vi "Accurate Measure With Setting - 複製.vi"(0 "DMM ref in":refnum<visa-resource-name>, 1 "channel_count":i32=11, 2 "P_current_count":i32, 3 "N_current_count":i32, 5 "DMM error in":errorcluster, 7 "Accurate Measure Setting":T1, 9 "ESP32 ref in":refnum<visa-resource-name>, 11 "ESP32 error in":errorcluster, 12 "current_mode":u8[](array[numeric])=[0, 0, 0, 0, 0, 0, 0, 0, 0, 0, 0]) -> (4 "DMM ref out":refnum<visa-resource-name>, 6 "DMM error out":errorcluster, 8 "Accurate Data":dbl[](array[numeric]), 10 "ESP32 ref out":refnum<visa-resource-name>, 13 "time_out_count":i32, 14 "Standard Deviation of Data":dbl[](array[numeric]), 15 "ESP32 error out":errorcluster)   [LabVIEW 2023]
uses:
  <instrlib>/Agilent 3446X Series/Agilent 3446X Series.lvlib
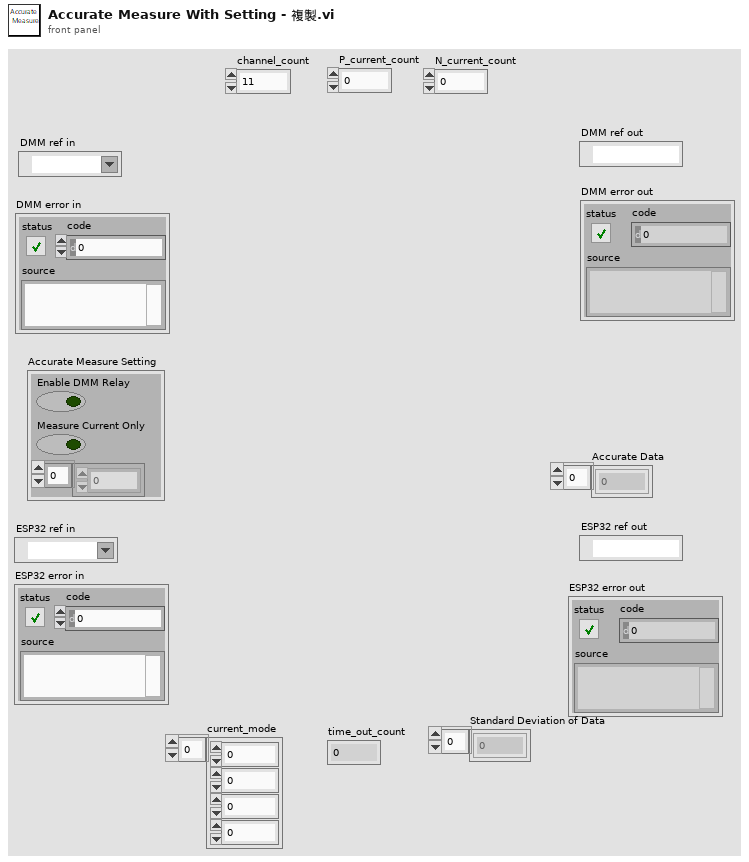
[diagram p1: front panel]
types:
  T1 = cluster{"Enable DMM Relay":bool, "Measure Current Only":bool, dbl[]}
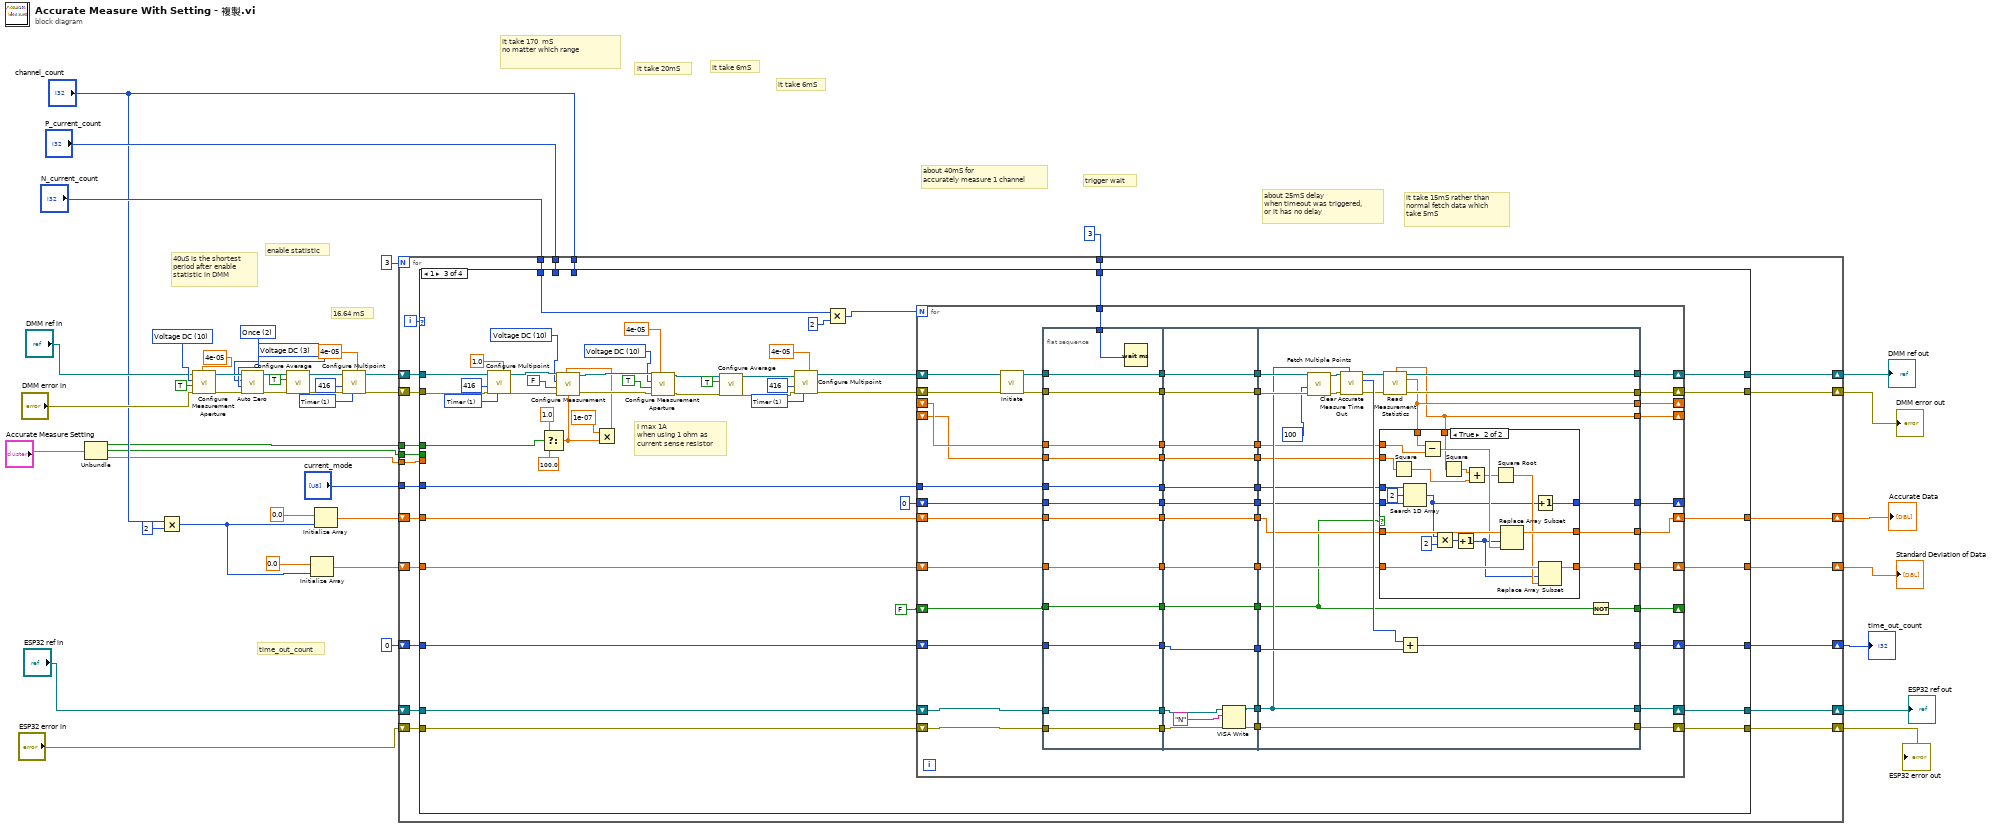
[diagram p0: block diagram]
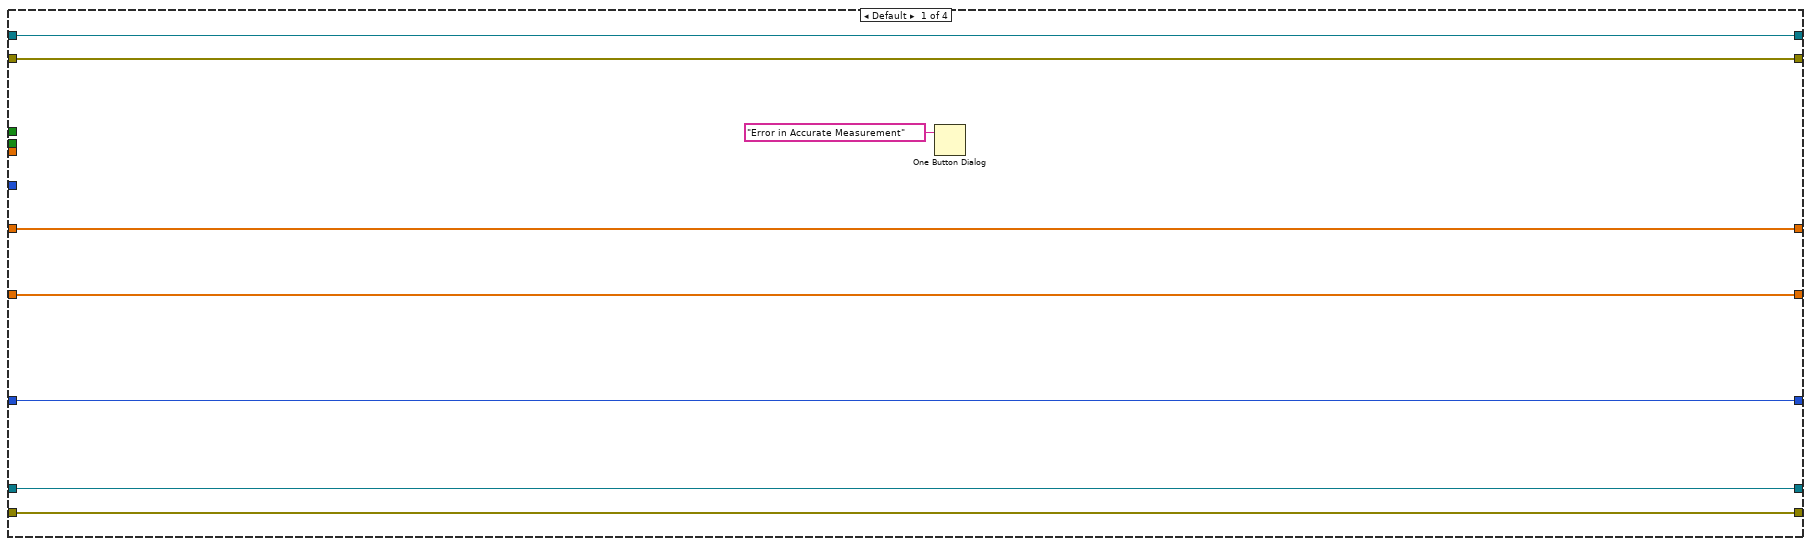
[diagram p2: hidden frame]
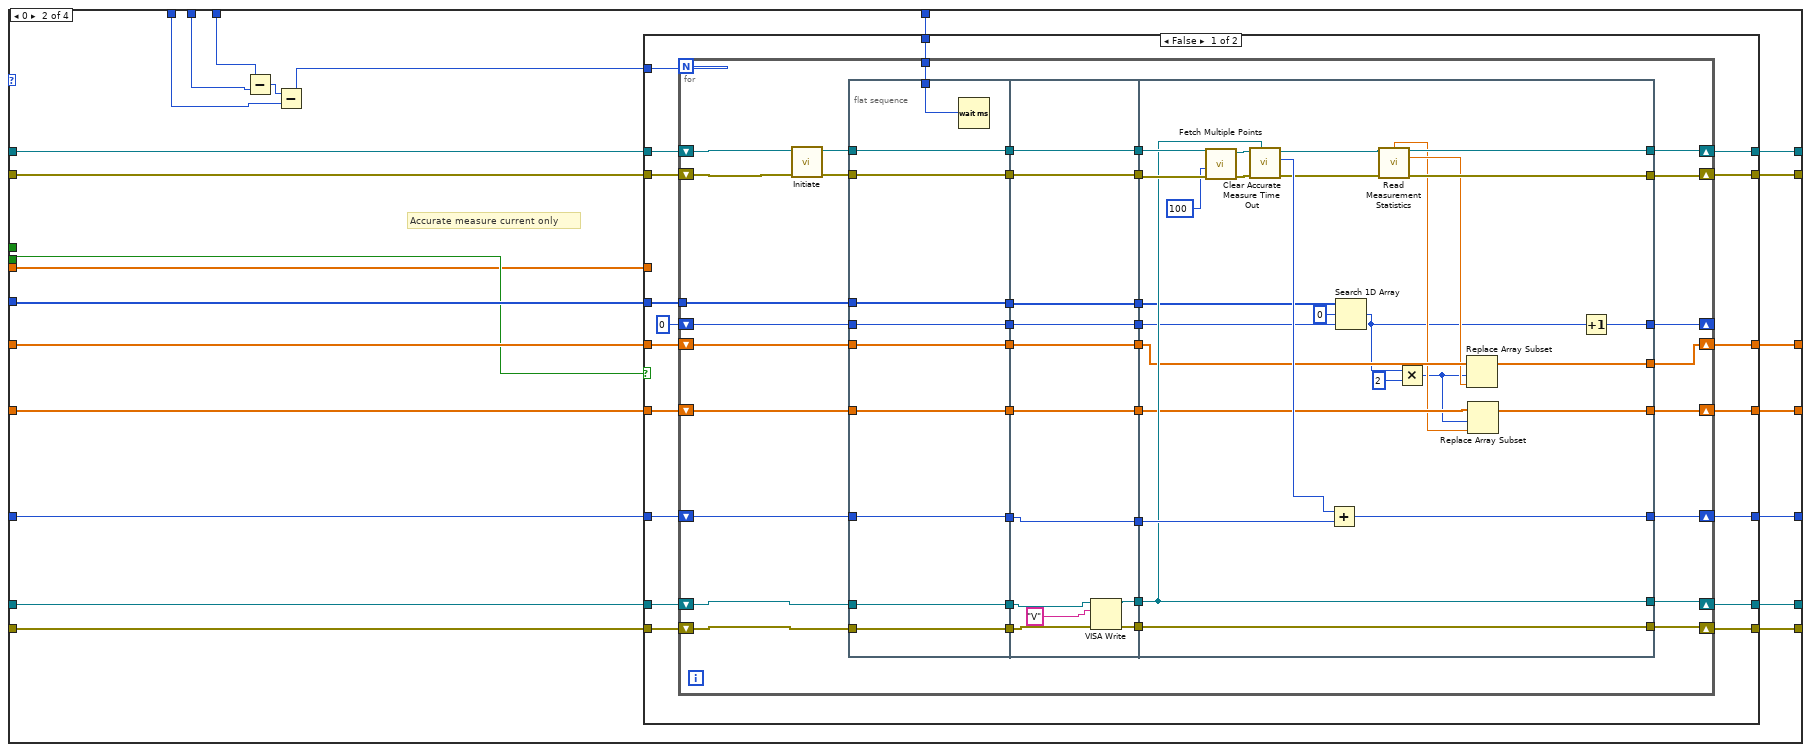
[diagram p3: hidden frame]
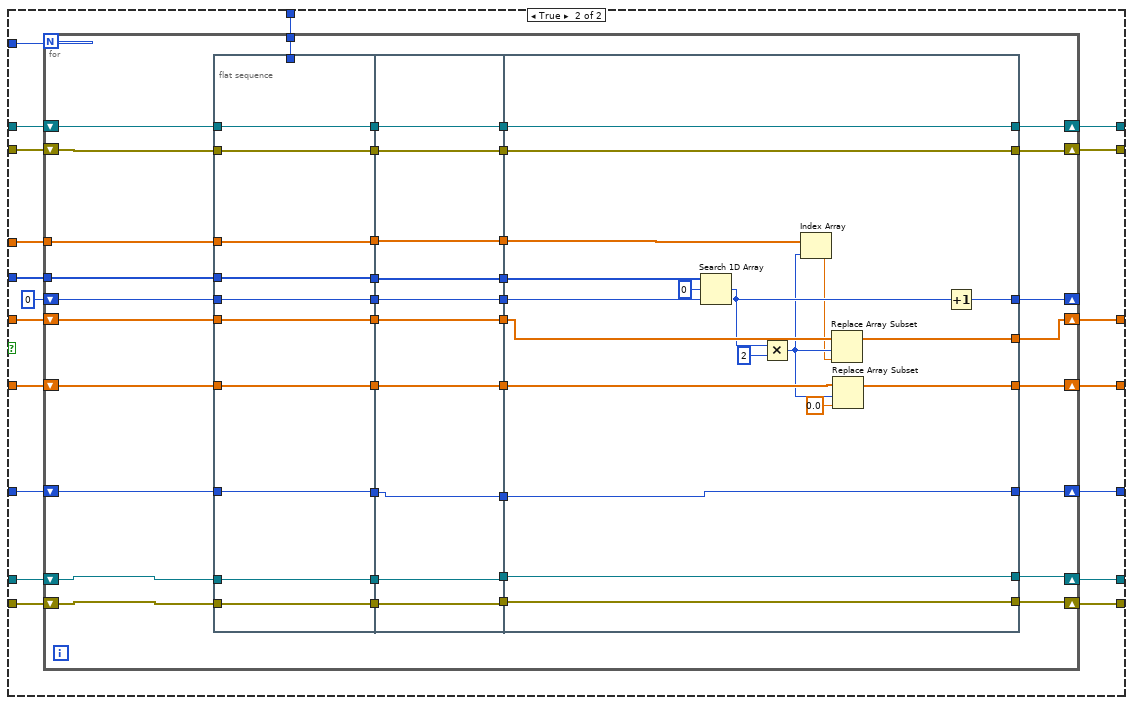
[diagram p4: hidden frame]
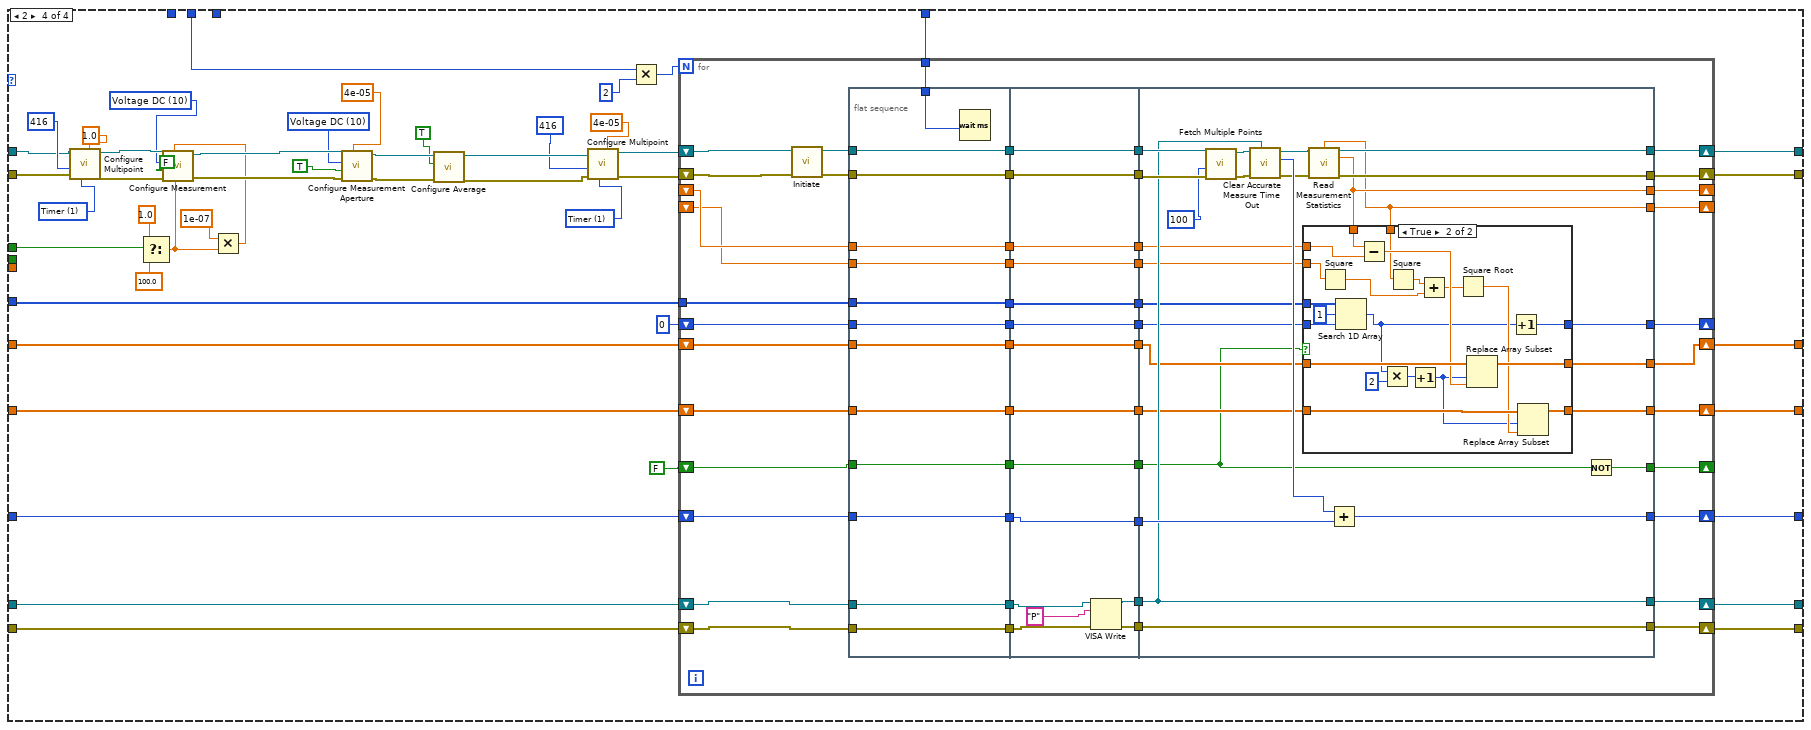
[diagram p6: hidden frame]
diagram:
  w32 = 1 items=["Immediate", "Timer"] ("Sample Source (0: Immediate)")
  w39 = 3 items=["Current DC", "Resistance", "Temperature", "Voltage DC"] ("Zero Type (0: Current DC)")
  w40 = 2 items=["Disable", "Enable", "Once"] ("Auto Zero (1: Enable)")
  w36 = 10 items=["Continuity", "Current AC", "Current DC", "Diode", "Frequency", "Resistance 4-wire", "Period", "Resistance 2-wire", "Temperature", "Voltage AC", "Voltage DC", "Voltage DC Ratio", "Capacitance"] ("Measurement Function (0: Continuity)")
  # "it take 6mS"
  # "it take 6mS"
  # "it take 20mS"
  # "it take 170  mS\nno matter which range"
  # "it take 15mS rather than\nnormal fetch data which \ntake 5mS"
  # "about 40mS for \naccurately measure 1 channel"
  # "about 25mS delay\nwhen timeout was triggered,\nor it has no delay"
  # "time_out_count"
  # "trigger wait"
  # "16.64 mS"
  # "enable statistic"
  # "40uS is the shortest\nperiod after enable \nstatistic in DMM"
  n1 = Unbundle("Accurate Measure Setting") -> ("Enable DMM Relay"=w4:bool, "Measure Current Only"=w2:bool, w1:dbl[])
  n2 = Multiply(x="channel_count", y=2) -> (x*y=w5:i32)
  n3 = call <instrlib>:"Configure Measurement Aperture.vi"("Aperture Time (0.1s)"=4e-05, "error in (no error)"="DMM error in", "Enable Aperture (F: Disable)"=TRUE, "Measurement Function (0: Continuity)"=w36, "VISA resource name"="DMM ref in") -> ("error out"=w43:errorcluster, "VISA resource name out"=w42:refnum<visa-resource-name>)  [unwired: 5 in]
  n4 = call <instrlib>:"Auto Zero.vi"("error in (no error)"=w43, "Auto Zero (1: Enable)"=w40, "Zero Type (0: Current DC)"=w39, "VISA resource name"=w42) -> ("error out"=w45:errorcluster, "VISA resource name out"=w44:refnum<visa-resource-name>)  [unwired: 6 in]
  n5 = call <instrlib>:"Configure Average.vi"("error in (no error)"=w45, "Enable Statistics (F: Disable)"=TRUE, "VISA resource name"=w44) -> ("error out"=w34:errorcluster, "VISA resource name out"=w35:refnum<visa-resource-name>)  [unwired: 7 in]
  n6 = Initialize Array(0.0 ("Arithmetic Mean"), w5) -> (w15:dbl[])
  n7 = Initialize Array(0.0 ("Arithmetic Mean"), w5) -> (w18:dbl[])
  n8 = call <instrlib>:"Configure Multipoint.vi"("Sample Interval (1 Second)"=4e-05, "Sample Source (0: Immediate)"=w32, "error in (no error)"=w34, "Sample Count (1)"=416, "VISA resource name"=w35) -> ("error out"=w29:errorcluster, "VISA resource name out"=w30:refnum<visa-resource-name>)  [unwired: 2 in, 3 out]
  n9 = for {
    N: 3 -> [_]
    shift-right: [w66] -> w11
    shift-left: "ESP32 ref in" -> [w68]
    shift-right: [w65] -> w10
    shift-left: "ESP32 error in" -> [w67]
    shift-right: [w62] -> w13
    shift-left: w30 -> [w64]
    shift-right: [w61] -> w12
    shift-left: w29 -> [w63]
    tunnel: "channel_count" -> [w60]
    tunnel: "P_current_count" -> [w59]
    tunnel: "N_current_count" -> [w58]
    tunnel: u32 3 ("milliseconds to wait") -> [w57]
    shift-right: [w56] -> w20
    shift-left: 0 -> [w55]
    shift-right: [w49] -> w9
    shift-left: w18 -> [w54]
    tunnel: "current_mode" -> [w53]
    shift-right: [w50] -> w8
    shift-left: w15 -> [w51]
    tunnel: w4 -> [w48]
    tunnel: w2 -> [w47]
    tunnel: w1 -> [w46]
    i -> [w52]
    n10 = case shown="1" w52 {
      tunnel: w68 -> [w74 w95 w350 w528]
      tunnel: w67 -> [w73 w94 w349 w527]
      tunnel: [w74 w91 w346 w524] -> w66
      tunnel: [w73 w90 w345 w523] -> w65
      tunnel: w64 -> [w76 w97 w314 w485]
      tunnel: w63 -> [w75 w96 w313 w484]
      tunnel: [w76 w93 w348 w526] -> w62
      tunnel: [w75 w92 w347 w525] -> w61
      tunnel: w60 -> [_ w89 _ _]
      tunnel: w59 -> [_ w88 _ w481]
      tunnel: w58 -> [_ w87 w309 _]
      tunnel: [w70 w85 w343 w521] -> w56
      tunnel: w57 -> [_ w86 w344 w522]
      tunnel: w55 -> [w70 w84 w342 w520]
      tunnel: w54 -> [w72 w82 w340 w518]
      tunnel: w53 -> [_ w83 w341 w519]
      tunnel: w51 -> [w71 w81 w338 w516]
      tunnel: [w71 w80 w337 w515] -> w50
      tunnel: [w72 w79 w336 w514] -> w49
      tunnel: w48 -> [_ _ w302 w486]
      tunnel: w47 -> [_ w78 _ _]
      tunnel: w46 -> [_ w77 _ _]
      frame Default {
        n11 = One Button Dialog(message="Error in Accurate Measurement") -> ()  [unwired: 1 in, 1 out]
      }
      frame 0 {
        # "Accurate measure current only"
        n12 = Subtract(x=w89, y=w88) -> (x-y=w99:i32)
        n13 = Subtract(x=w99, y=w87) -> (x-y=w98:i32)
        n14 = case shown="False" w78 {
          tunnel: w98 -> [w117 w223]
          tunnel: w97 -> [w116 w222]
          tunnel: w96 -> [w115 w221]
          tunnel: w95 -> [w114 w220]
          tunnel: w94 -> [w113 w219]
          tunnel: [w112 w218] -> w93
          tunnel: [w111 w217] -> w92
          tunnel: [w110 w216] -> w91
          tunnel: [w109 w215] -> w90
          tunnel: w86 -> [w108 w214]
          tunnel: [w107 w213] -> w85
          tunnel: w84 -> [w106 w212]
          tunnel: w83 -> [w105 w211]
          tunnel: w82 -> [w104 w210]
          tunnel: w81 -> [w102 w208]
          tunnel: [w101 w207] -> w80
          tunnel: [w100 w206] -> w79
          tunnel: w77 -> [_ w205]
          frame False {
            n15 = for {
              N: w117 -> [_]
              shift-right: [w151] -> w112
              shift-left: w116 -> [w155]
              shift-right: [w150] -> w111
              shift-left: w115 -> [w154]
              shift-right: [w149] -> w110
              shift-left: w114 -> [w153]
              shift-right: [w148] -> w109
              shift-left: w113 -> [w152]
              tunnel: w108 -> [w134]
              shift-right: [w133] -> w107
              shift-left: w106 -> [w147]
              tunnel: w105 -> [w131]
              shift-right: [w119] -> w100
              shift-left: w104 -> [w128]
              shift-right: [w123] -> _
              shift-left: 0 ("index of element") -> [w124]
              shift-right: [w118] -> w101
              shift-left: w102 -> [w121]
              n16 = call <instrlib>:"Initiate.vi"("error in (no error)"=w154, "VISA resource name"=w155) -> ("error out"=w135:errorcluster, "VISA resource name out"=w136:refnum<visa-resource-name>)  [unwired: 8 in]
              n17 = flat-sequence {
                tunnel: [w165] -> w146
                tunnel: w153 -> [w165]
                tunnel: [w164] -> w145
                tunnel: w152 -> [w164]
                tunnel: w136 -> [w163]
                tunnel: [w163] -> w144
                tunnel: [w162] -> w143
                tunnel: w135 -> [w162]
                tunnel: [w161] -> w142
                tunnel: w147 -> [w161]
                tunnel: w134 -> [w160]
                tunnel: [w159] -> w132
                tunnel: w131 -> [w159]
                tunnel: [w158] -> w129
                tunnel: w128 -> [w158]
                tunnel: w124 -> [w157]
                tunnel: [w157] -> w126
                tunnel: [w156] -> w122
                tunnel: w121 -> [w156]
                tunnel: w146 -> [w177]
                tunnel: w145 -> [w176]
                tunnel: w144 -> [w175]
                tunnel: [w175] -> w138
                tunnel: w143 -> [w174]
                tunnel: [w174] -> w139
                tunnel: [w173] -> w140
                tunnel: [w172] -> w141
                tunnel: w142 -> [w170]
                tunnel: [w170] -> w137
                tunnel: w132 -> [w169]
                tunnel: [w169] -> w130
                tunnel: w129 -> [w168]
                tunnel: [w168] -> w127
                tunnel: w126 -> [w167]
                tunnel: [w167] -> w125
                tunnel: w122 -> [w166]
                tunnel: [w166] -> w120
                tunnel: [w204] -> w148
                tunnel: [w192] -> w149
                tunnel: [w196] -> w150
                tunnel: [w197] -> w151
                tunnel: w141 -> [w204]
                tunnel: w140 -> [w192]
                tunnel: w139 -> [w203]
                tunnel: w138 -> [w202]
                tunnel: [w198] -> w133
                tunnel: w137 -> [w193]
                tunnel: w130 -> [w191]
                tunnel: w127 -> [w187]
                tunnel: w125 -> [w189]
                tunnel: [w188] -> w123
                tunnel: w120 -> [w185]
                tunnel: [w183] -> w119
                tunnel: [w182] -> w118
                frame #0 {
                  n18 = Wait (ms)(milliseconds to wait=w160) -> ()  [unwired: 1 out]
                }
                frame #1 {
                  n19 = VISA Write(VISA resource name=w177, write buffer="V" ("data in"), error in (no error)=w176) -> (VISA resource name out=w173:refnum<visa-resource-name>, error out=w172:errorcluster)  [unwired: 1 out]
                }
                frame #2 {
                  n20 = call <instrlib>:"Fetch Multiple Points.vi"("error in (no error)"=w203, "Timeout (10000 ms)"=100, "VISA resource name"=w202) -> ("error out"=w200:errorcluster, "VISA resource name out"=w201:refnum<visa-resource-name>)  [unwired: 1 in, 6 out]
                  n21 = call "Clear Accurate Measure Time Out.vi"("ESP32 ref"=w192, "error in (no error)"=w200, "DMM ref"=w201) -> ("error out"=w194:errorcluster, "Time out count"=w199:i32, "VISA Refnum out"=w195:refnum<visa-resource-name>)  [unwired: 5 in, 1 out]
                  n22 = Add(x=w199, y=w193) -> (x+y=w198:i32)
                  n23 = Search 1D Array(1D array=w191, element=u8 0, start index (0)=w189) -> (index of element=w180:i32)
                  n24 = call <instrlib>:"Read Measurement Statistics.vi"("VISA resource name"=w195, "error in (no error)"=w194) -> ("Standard Deviation"=w184:dbl, "VISA resource name out"=w197:refnum<visa-resource-name>, "Arithmetic Mean"=w186:dbl, "error out"=w196:errorcluster)  [unwired: 6 in, 4 out]
                  n25 = Multiply(x=w180, y=2) -> (x*y=w178:i32)
                  n26 = Replace Array Subset(array=w187, new element=w186, index=w178) -> (w183:dbl[])
                  n27 = Replace Array Subset(array=w185, new element=w184, index=w178) -> (w182:dbl[])
                  n28 = Increment(x=w180) -> (x+1=w188:i32)
                }
              }
            }
          }
          frame True {
            n29 = for {
              N: w223 -> [_]
              shift-right: [w232] -> w218
              shift-left: w222 -> [w234]
              shift-right: [w227] -> w217
              shift-left: w221 -> [w229]
              shift-right: [w260] -> w216
              shift-left: w220 -> [w262]
              shift-right: [w259] -> w215
              shift-left: w219 -> [w261]
              tunnel: w214 -> [w251]
              shift-right: [w250] -> w213
              shift-left: w212 -> [w258]
              tunnel: w211 -> [w248]
              shift-right: [w236] -> w206
              shift-left: w210 -> [w245]
              shift-right: [w240] -> _
              shift-left: 0 ("index of element") -> [w241]
              shift-right: [w235] -> w207
              shift-left: w208 -> [w238]
              tunnel: w205 -> [w224]
              n30 = flat-sequence {
                tunnel: [w272] -> w257
                tunnel: w262 -> [w272]
                tunnel: [w271] -> w256
                tunnel: w261 -> [w271]
                tunnel: [w270] -> w255
                tunnel: w258 -> [w270]
                tunnel: w251 -> [_]
                tunnel: [w269] -> w249
                tunnel: w248 -> [w269]
                tunnel: [w268] -> w246
                tunnel: w245 -> [w268]
                tunnel: w241 -> [w267]
                tunnel: [w267] -> w243
                tunnel: [w266] -> w239
                tunnel: w238 -> [w266]
                tunnel: w234 -> [w265]
                tunnel: [w265] -> w231
                tunnel: [w264] -> w230
                tunnel: w229 -> [w264]
                tunnel: [w263] -> w226
                tunnel: w224 -> [w263]
                tunnel: w257 -> [w275]
                tunnel: w256 -> [w274]
                tunnel: [w275] -> w253
                tunnel: [w274] -> w254
                tunnel: w255 -> [w282]
                tunnel: [w282] -> w252
                tunnel: w249 -> [w281]
                tunnel: [w281] -> w247
                tunnel: w246 -> [w280]
                tunnel: [w280] -> w244
                tunnel: w243 -> [w279]
                tunnel: [w279] -> w242
                tunnel: w239 -> [w278]
                tunnel: [w278] -> w237
                tunnel: [w277] -> w233
                tunnel: w231 -> [w277]
                tunnel: w230 -> [w276]
                tunnel: [w276] -> w228
                tunnel: w226 -> [w273]
                tunnel: [w273] -> w225
                tunnel: [w301] -> w259
                tunnel: [w300] -> w260
                tunnel: w254 -> [w301]
                tunnel: w253 -> [w300]
                tunnel: [w283] -> w250
                tunnel: w252 -> [w283]
                tunnel: w247 -> [w299]
                tunnel: w244 -> [w295]
                tunnel: w242 -> [w297]
                tunnel: [w296] -> w240
                tunnel: w237 -> [w294]
                tunnel: [w293] -> w236
                tunnel: [w292] -> w235
                tunnel: w233 -> [w289]
                tunnel: [w289] -> w232
                tunnel: [w288] -> w227
                tunnel: w228 -> [w288]
                tunnel: w225 -> [w286]
                frame #0 {
                }
                frame #1 {
                }
                frame #2 {
                  n31 = Search 1D Array(1D array=w299, element=u8 0, start index (0)=w297) -> (index of element=w291:i32)
                  n32 = Multiply(x=w291, y=2) -> (x*y=w285:i32)
                  n33 = Index Array(array=w286, index=w285) -> (element=w284:dbl)
                  n34 = Replace Array Subset(array=w295, new element=w284, index=w285) -> (w293:dbl[])
                  n35 = Replace Array Subset(array=w294, new element=0.0 ("new element/subarray"), index=w285) -> (w292:dbl[])
                  n36 = Increment(x=w291) -> (x+1=w296:i32)
                }
              }
            }
          }
        }
      }
      frame 1 {
        w325 = 1 items=["Immediate", "Timer"] ("Sample Source (0: Immediate)")
        w321 = 10 items=["Continuity", "Current AC", "Current DC", "Diode", "Frequency", "Resistance 4-wire", "Period", "Resistance 2-wire", "Temperature", "Voltage AC", "Voltage DC", "Voltage DC Ratio", "Capacitance"] ("Measurement Function (0: Continuity)")
        w318 = 1 items=["Immediate", "Timer"] ("Sample Source (0: Immediate)")
        w315 = 10 items=["Continuity", "Current AC", "Current DC", "Diode", "Frequency", "Resistance 4-wire", "Period", "Resistance 2-wire", "Temperature", "Voltage AC", "Voltage DC", "Voltage DC Ratio", "Capacitance"] ("Measurement Function (10: Voltage DC)")
        # "I max 1A\nwhen using 1 ohm as \ncurrent sense resistor"
        n37 = call <instrlib>:"Configure Multipoint.vi"("Sample Interval (1 Second)"=1.0, "Sample Source (0: Immediate)"=w318, "error in (no error)"=w313, "Sample Count (1)"=416, "VISA resource name"=w314) -> ("error out"=w332:errorcluster, "VISA resource name out"=w331:refnum<visa-resource-name>)  [unwired: 2 in, 3 out]
        n38 = Select(t=1.0 ("Manual Range (1)"), s=w302, f=100.0 ("Manual Range (1)")) -> (s? t:f=w304:dbl)
        n39 = Multiply(x=1e-07, y=w304) -> (x*y=w303:dbl)
        n40 = call <instrlib>:"Configure Measurement.vi"("Manual Range (1)"=w304, "Absolute Resolution (1E-6)"=w303, "error in (no error)"=w332, "Auto Range (T: Enable)"=FALSE, "Measurement Function (10: Voltage DC)"=w315, "VISA resource name"=w331) -> ("error out"=w329:errorcluster, "VISA resource name out"=w330:refnum<visa-resource-name>)  [unwired: 4 out]
        n41 = call <instrlib>:"Configure Measurement Aperture.vi"("Aperture Time (0.1s)"=4e-05, "error in (no error)"=w329, "Enable Aperture (F: Disable)"=TRUE, "Measurement Function (0: Continuity)"=w321, "VISA resource name"=w330) -> ("error out"=w334:errorcluster, "VISA resource name out"=w335:refnum<visa-resource-name>)  [unwired: 5 in]
        n42 = call <instrlib>:"Configure Average.vi"("error in (no error)"=w334, "Enable Statistics (F: Disable)"=TRUE, "VISA resource name"=w335) -> ("error out"=w333:errorcluster, "VISA resource name out"=w328:refnum<visa-resource-name>)  [unwired: 7 in]
        n43 = call <instrlib>:"Configure Multipoint.vi"("Sample Interval (1 Second)"=4e-05, "Sample Source (0: Immediate)"=w325, "error in (no error)"=w333, "Sample Count (1)"=416, "VISA resource name"=w328) -> ("error out"=w311:errorcluster, "VISA resource name out"=w312:refnum<visa-resource-name>)  [unwired: 2 in, 3 out]
        n44 = Multiply(x=w309, y=2) -> (x*y=w310:i32)
        n45 = for {
          N: w310 -> [_]
          shift-right: [w396] -> w348
          shift-left: w312 -> [w400]
          shift-right: [w395] -> w347
          shift-left: w311 -> [w399]
          shift-right: [w394] -> w346
          shift-left: w350 -> [w398]
          shift-right: [w393] -> w345
          shift-left: w349 -> [w397]
          tunnel: w344 -> [w379]
          shift-right: [w378] -> w343
          shift-left: w342 -> [w392]
          tunnel: w341 -> [w376]
          shift-right: [w364] -> w336
          shift-left: w340 -> [w373]
          shift-right: [w368] -> _
          shift-left: 0 ("index of element") -> [w369]
          shift-right: [w363] -> w337
          shift-left: w338 -> [w366]
          shift-right: [w359] -> _
          shift-left: FALSE ("Enable Statistics (F: Disable)") -> [w360]
          shift-right: [w358] -> _
          shift-left: _ -> [w356]
          shift-right: [w357] -> _
          shift-left: _ -> [w353]
          n46 = call <instrlib>:"Initiate.vi"("error in (no error)"=w399, "VISA resource name"=w400) -> ("error out"=w380:errorcluster, "VISA resource name out"=w381:refnum<visa-resource-name>)  [unwired: 8 in]
          n47 = flat-sequence {
            tunnel: [w413] -> w391
            tunnel: w398 -> [w413]
            tunnel: [w412] -> w390
            tunnel: w397 -> [w412]
            tunnel: w381 -> [w411]
            tunnel: [w411] -> w389
            tunnel: [w410] -> w388
            tunnel: w380 -> [w410]
            tunnel: [w409] -> w387
            tunnel: w392 -> [w409]
            tunnel: w379 -> [w408]
            tunnel: [w407] -> w377
            tunnel: w376 -> [w407]
            tunnel: [w406] -> w374
            tunnel: w373 -> [w406]
            tunnel: w369 -> [w405]
            tunnel: [w405] -> w371
            tunnel: [w404] -> w367
            tunnel: w366 -> [w404]
            tunnel: w360 -> [w403]
            tunnel: [w403] -> w362
            tunnel: w356 -> [w402]
            tunnel: [w402] -> w354
            tunnel: w353 -> [w401]
            tunnel: [w401] -> w352
            tunnel: w391 -> [w428]
            tunnel: w390 -> [w427]
            tunnel: w389 -> [w426]
            tunnel: [w426] -> w383
            tunnel: w388 -> [w425]
            tunnel: [w425] -> w384
            tunnel: [w424] -> w385
            tunnel: [w423] -> w386
            tunnel: w387 -> [w421]
            tunnel: [w421] -> w382
            tunnel: w377 -> [w420]
            tunnel: [w420] -> w375
            tunnel: w374 -> [w419]
            tunnel: [w419] -> w372
            tunnel: w371 -> [w418]
            tunnel: [w418] -> w370
            tunnel: w367 -> [w417]
            tunnel: [w417] -> w365
            tunnel: w362 -> [w416]
            tunnel: [w416] -> w361
            tunnel: [w415] -> w355
            tunnel: w354 -> [w415]
            tunnel: w352 -> [w414]
            tunnel: [w414] -> w351
            tunnel: [w455] -> w393
            tunnel: [w443] -> w394
            tunnel: [w447] -> w395
            tunnel: [w448] -> w396
            tunnel: w386 -> [w455]
            tunnel: w385 -> [w443]
            tunnel: w384 -> [w454]
            tunnel: w383 -> [w453]
            tunnel: [w449] -> w378
            tunnel: w382 -> [w444]
            tunnel: w375 -> [w442]
            tunnel: w372 -> [w439]
            tunnel: w370 -> [w441]
            tunnel: [w440] -> w368
            tunnel: w365 -> [w438]
            tunnel: [w437] -> w364
            tunnel: [w436] -> w363
            tunnel: w361 -> [w435]
            tunnel: [w434] -> w359
            tunnel: [w431] -> w358
            tunnel: [w430] -> w357
            tunnel: w355 -> [w433]
            tunnel: w351 -> [w432]
            frame #0 {
              n48 = Wait (ms)(milliseconds to wait=w408) -> ()  [unwired: 1 out]
            }
            frame #1 {
              n49 = VISA Write(VISA resource name=w428, write buffer="N" ("data in"), error in (no error)=w427) -> (VISA resource name out=w424:refnum<visa-resource-name>, error out=w423:errorcluster)  [unwired: 1 out]
            }
            frame #2 {
              n50 = call <instrlib>:"Fetch Multiple Points.vi"("error in (no error)"=w454, "Timeout (10000 ms)"=100, "VISA resource name"=w453) -> ("error out"=w451:errorcluster, "VISA resource name out"=w452:refnum<visa-resource-name>)  [unwired: 1 in, 6 out]
              n51 = call "Clear Accurate Measure Time Out.vi"("ESP32 ref"=w443, "error in (no error)"=w451, "DMM ref"=w452) -> ("error out"=w445:errorcluster, "Time out count"=w450:i32, "VISA Refnum out"=w446:refnum<visa-resource-name>)  [unwired: 5 in, 1 out]
              n52 = call <instrlib>:"Read Measurement Statistics.vi"("VISA resource name"=w446, "error in (no error)"=w445) -> ("Standard Deviation"=w430:dbl, "VISA resource name out"=w448:refnum<visa-resource-name>, "Arithmetic Mean"=w431:dbl, "error out"=w447:errorcluster)  [unwired: 6 in, 4 out]
              n53 = case shown="True" w435 {
                tunnel: w442 -> [_ w479]
                tunnel: w441 -> [w458 w477]
                tunnel: [w458 w476] -> w440
                tunnel: w439 -> [w457 w475]
                tunnel: w438 -> [w456 w474]
                tunnel: [w457 w473] -> w437
                tunnel: [w456 w472] -> w436
                tunnel: w433 -> [_ w463]
                tunnel: w432 -> [_ w470]
                tunnel: w431 -> [_ w464]
                tunnel: w430 -> [_ w469]
                frame False {
                }
                frame True {
                  n54 = Square(x=w470) -> (x^2=w467:dbl)
                  n55 = Search 1D Array(1D array=w479, element=u8 2, start index (0)=w477) -> (index of element=w460:i32)
                  n56 = Subtract(x=w464, y=w463) -> (x-y=w471:dbl)
                  n57 = Multiply(x=w460, y=2) -> (x*y=w461:i32)
                  n58 = Square(x=w469) -> (x^2=w468:dbl)
                  n59 = Increment(x=w461) -> (x+1=w459:i32)
                  n60 = Add(x=w468, y=w467) -> (x+y=w466:dbl)
                  n61 = Square Root(x=w466) -> (sqrt(x)=w465:dbl)
                  n62 = Replace Array Subset(array=w475, new element=w471, index=w459) -> (w473:dbl[])
                  n63 = Increment(x=w460) -> (x+1=w476:i32)
                  n64 = Replace Array Subset(array=w474, new element=w465, index=w459) -> (w472:dbl[])
                }
              }
              n65 = Add(x=w450, y=w444) -> (x+y=w449:i32)
              n66 = Not(x=w435) -> (.not. x?=w434:bool)
            }
          }
        }
      }
      frame 2 {
        w500 = 1 items=["Immediate", "Timer"] ("Sample Source (0: Immediate)")
        w496 = 10 items=["Continuity", "Current AC", "Current DC", "Diode", "Frequency", "Resistance 4-wire", "Period", "Resistance 2-wire", "Temperature", "Voltage AC", "Voltage DC", "Voltage DC Ratio", "Capacitance"] ("Measurement Function (0: Continuity)")
        w493 = 1 items=["Immediate", "Timer"] ("Sample Source (0: Immediate)")
        w490 = 10 items=["Continuity", "Current AC", "Current DC", "Diode", "Frequency", "Resistance 4-wire", "Period", "Resistance 2-wire", "Temperature", "Voltage AC", "Voltage DC", "Voltage DC Ratio", "Capacitance"] ("Measurement Function (10: Voltage DC)")
        n67 = call <instrlib>:"Configure Multipoint.vi"("Sample Interval (1 Second)"=1.0, "Sample Source (0: Immediate)"=w493, "error in (no error)"=w484, "Sample Count (1)"=416, "VISA resource name"=w485) -> ("error out"=w509:errorcluster, "VISA resource name out"=w508:refnum<visa-resource-name>)  [unwired: 2 in, 3 out]
        n68 = Select(t=1.0 ("Manual Range (1)"), s=w486, f=100.0 ("Manual Range (1)")) -> (s? t:f=w489:dbl)
        n69 = Multiply(x=1e-07, y=w489) -> (x*y=w488:dbl)
        n70 = call <instrlib>:"Configure Measurement.vi"("Manual Range (1)"=w489, "Absolute Resolution (1E-6)"=w488, "error in (no error)"=w509, "Auto Range (T: Enable)"=FALSE, "Measurement Function (10: Voltage DC)"=w490, "VISA resource name"=w508) -> ("error out"=w506:errorcluster, "VISA resource name out"=w507:refnum<visa-resource-name>)  [unwired: 4 out]
        n71 = call <instrlib>:"Configure Measurement Aperture.vi"("Aperture Time (0.1s)"=4e-05, "error in (no error)"=w506, "Enable Aperture (F: Disable)"=TRUE, "Measurement Function (0: Continuity)"=w496, "VISA resource name"=w507) -> ("error out"=w511:errorcluster, "VISA resource name out"=w512:refnum<visa-resource-name>)  [unwired: 5 in]
        n72 = call <instrlib>:"Configure Average.vi"("error in (no error)"=w511, "Enable Statistics (F: Disable)"=TRUE, "VISA resource name"=w512) -> ("error out"=w510:errorcluster, "VISA resource name out"=w505:refnum<visa-resource-name>)  [unwired: 7 in]
        n73 = call <instrlib>:"Configure Multipoint.vi"("Sample Interval (1 Second)"=4e-05, "Sample Source (0: Immediate)"=w500, "error in (no error)"=w510, "Sample Count (1)"=416, "VISA resource name"=w505) -> ("error out"=w482:errorcluster, "VISA resource name out"=w483:refnum<visa-resource-name>)  [unwired: 2 in, 3 out]
        n74 = Multiply(x=w481, y=2) -> (x*y=w480:i32)
        n75 = for {
          N: w480 -> [_]
          shift-right: [w574] -> w526
          shift-left: w483 -> [w578]
          shift-right: [w573] -> w525
          shift-left: w482 -> [w577]
          shift-right: [w572] -> w524
          shift-left: w528 -> [w576]
          shift-right: [w571] -> w523
          shift-left: w527 -> [w575]
          tunnel: w522 -> [w557]
          shift-right: [w556] -> w521
          shift-left: w520 -> [w570]
          tunnel: w519 -> [w554]
          shift-right: [w542] -> w514
          shift-left: w518 -> [w551]
          shift-right: [w546] -> _
          shift-left: 0 ("index of element") -> [w547]
          shift-right: [w541] -> w515
          shift-left: w516 -> [w544]
          shift-right: [w537] -> _
          shift-left: FALSE ("Enable Statistics (F: Disable)") -> [w538]
          shift-right: [w536] -> _
          shift-left: _ -> [w534]
          shift-right: [w535] -> _
          shift-left: _ -> [w531]
          n76 = call <instrlib>:"Initiate.vi"("error in (no error)"=w577, "VISA resource name"=w578) -> ("error out"=w558:errorcluster, "VISA resource name out"=w559:refnum<visa-resource-name>)  [unwired: 8 in]
          n77 = flat-sequence {
            tunnel: [w591] -> w569
            tunnel: w576 -> [w591]
            tunnel: [w590] -> w568
            tunnel: w575 -> [w590]
            tunnel: w559 -> [w589]
            tunnel: [w589] -> w567
            tunnel: [w588] -> w566
            tunnel: w558 -> [w588]
            tunnel: [w587] -> w565
            tunnel: w570 -> [w587]
            tunnel: w557 -> [w586]
            tunnel: [w585] -> w555
            tunnel: w554 -> [w585]
            tunnel: [w584] -> w552
            tunnel: w551 -> [w584]
            tunnel: w547 -> [w583]
            tunnel: [w583] -> w549
            tunnel: [w582] -> w545
            tunnel: w544 -> [w582]
            tunnel: w538 -> [w581]
            tunnel: [w581] -> w540
            tunnel: w534 -> [w580]
            tunnel: [w580] -> w532
            tunnel: w531 -> [w579]
            tunnel: [w579] -> w530
            tunnel: w569 -> [w606]
            tunnel: w568 -> [w605]
            tunnel: w567 -> [w604]
            tunnel: [w604] -> w561
            tunnel: w566 -> [w603]
            tunnel: [w603] -> w562
            tunnel: [w602] -> w563
            tunnel: [w601] -> w564
            tunnel: w565 -> [w599]
            tunnel: [w599] -> w560
            tunnel: w555 -> [w598]
            tunnel: [w598] -> w553
            tunnel: w552 -> [w597]
            tunnel: [w597] -> w550
            tunnel: w549 -> [w596]
            tunnel: [w596] -> w548
            tunnel: w545 -> [w595]
            tunnel: [w595] -> w543
            tunnel: w540 -> [w594]
            tunnel: [w594] -> w539
            tunnel: [w593] -> w533
            tunnel: w532 -> [w593]
            tunnel: w530 -> [w592]
            tunnel: [w592] -> w529
            tunnel: [w633] -> w571
            tunnel: [w621] -> w572
            tunnel: [w625] -> w573
            tunnel: [w626] -> w574
            tunnel: w564 -> [w633]
            tunnel: w563 -> [w621]
            tunnel: w562 -> [w632]
            tunnel: w561 -> [w631]
            tunnel: [w627] -> w556
            tunnel: w560 -> [w622]
            tunnel: w553 -> [w620]
            tunnel: w550 -> [w617]
            tunnel: w548 -> [w619]
            tunnel: [w618] -> w546
            tunnel: w543 -> [w616]
            tunnel: [w615] -> w542
            tunnel: [w614] -> w541
            tunnel: w539 -> [w613]
            tunnel: [w612] -> w537
            tunnel: [w609] -> w536
            tunnel: [w608] -> w535
            tunnel: w533 -> [w611]
            tunnel: w529 -> [w610]
            frame #0 {
              n78 = Wait (ms)(milliseconds to wait=w586) -> ()  [unwired: 1 out]
            }
            frame #1 {
              n79 = VISA Write(VISA resource name=w606, write buffer="P" ("data in"), error in (no error)=w605) -> (VISA resource name out=w602:refnum<visa-resource-name>, error out=w601:errorcluster)  [unwired: 1 out]
            }
            frame #2 {
              n80 = call <instrlib>:"Fetch Multiple Points.vi"("error in (no error)"=w632, "Timeout (10000 ms)"=100, "VISA resource name"=w631) -> ("error out"=w629:errorcluster, "VISA resource name out"=w630:refnum<visa-resource-name>)  [unwired: 1 in, 6 out]
              n81 = call "Clear Accurate Measure Time Out.vi"("ESP32 ref"=w621, "error in (no error)"=w629, "DMM ref"=w630) -> ("error out"=w623:errorcluster, "Time out count"=w628:i32, "VISA Refnum out"=w624:refnum<visa-resource-name>)  [unwired: 5 in, 1 out]
              n82 = call <instrlib>:"Read Measurement Statistics.vi"("VISA resource name"=w624, "error in (no error)"=w623) -> ("Standard Deviation"=w608:dbl, "VISA resource name out"=w626:refnum<visa-resource-name>, "Arithmetic Mean"=w609:dbl, "error out"=w625:errorcluster)  [unwired: 6 in, 4 out]
              n83 = case shown="True" w613 {
                tunnel: w620 -> [_ w657]
                tunnel: w619 -> [w636 w655]
                tunnel: [w636 w654] -> w618
                tunnel: w617 -> [w635 w653]
                tunnel: w616 -> [w634 w652]
                tunnel: [w635 w651] -> w615
                tunnel: [w634 w650] -> w614
                tunnel: w611 -> [_ w641]
                tunnel: w610 -> [_ w648]
                tunnel: w609 -> [_ w642]
                tunnel: w608 -> [_ w647]
                frame False {
                }
                frame True {
                  n84 = Square(x=w648) -> (x^2=w645:dbl)
                  n85 = Search 1D Array(1D array=w657, element=u8 1, start index (0)=w655) -> (index of element=w638:i32)
                  n86 = Subtract(x=w642, y=w641) -> (x-y=w649:dbl)
                  n87 = Multiply(x=w638, y=2) -> (x*y=w639:i32)
                  n88 = Square(x=w647) -> (x^2=w646:dbl)
                  n89 = Increment(x=w639) -> (x+1=w637:i32)
                  n90 = Add(x=w646, y=w645) -> (x+y=w644:dbl)
                  n91 = Square Root(x=w644) -> (sqrt(x)=w643:dbl)
                  n92 = Replace Array Subset(array=w653, new element=w649, index=w637) -> (w651:dbl[])
                  n93 = Increment(x=w638) -> (x+1=w654:i32)
                  n94 = Replace Array Subset(array=w652, new element=w643, index=w637) -> (w650:dbl[])
                }
              }
              n95 = Add(x=w628, y=w622) -> (x+y=w627:i32)
              n96 = Not(x=w613) -> (.not. x?=w612:bool)
            }
          }
        }
      }
    }
  }
  "time_out_count" <- w20
  "DMM ref out" <- w13
  "DMM error out" <- w12
  "ESP32 ref out" <- w11
  "ESP32 error out" <- w10
  "Accurate Data" <- w9
  "Standard Deviation of Data" <- w8
